vi "Get Channel.vi"(9 "name":string, 10 "Gateway IP Address (\"\": localhost)":string, 11 "Sequence Context":refnum<k7>) -> (0 "error out":errorcluster, 2 "Channel.Unit":string, 3 "Channel.Value":dbl)   [LabVIEW 2013, in "Set Channels.lvlib"]
uses:
  Set Channels.lvlib
  <vilib>/NI Veristand/Execution/Workspace/NI VeriStand - Get Single Channel Value.vi
  <vilib>/NI Veristand/Execution/Workspace/NI_VS Workspace ExecutionAPI.lvlib
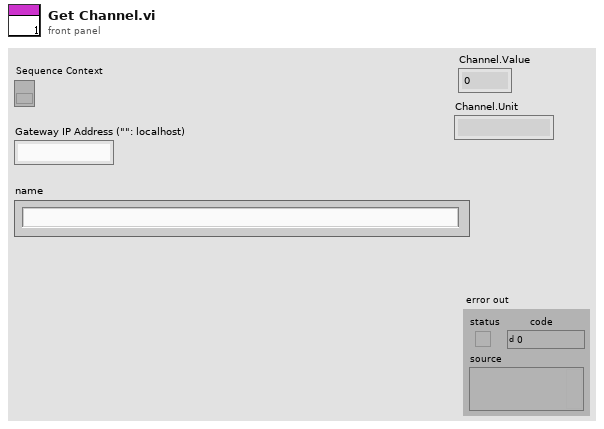
[diagram p1: front panel]
types:
  T1 = typedef "NI_VS Workspace ExecutionAPI.lvlib/WorkspaceAPI.ctl" = refnum<k24>
  T2 = typedef "NI_VS Workspace ExecutionAPI.lvlib/NodeInfo.ctl" = cluster{"Name":string, "FullPath":string, "Type":string, "IsChannel":bool, "Channel":cluster{"Unit":string, "Readable":bool, "Writable":bool, "Faultable":bool, "Scalable":bool, "RowDim":u32, "ColumnDim":u32}, "IsWaveform":bool, "Waveform":cluster{"DataType":T3}}
  T3 = typedef "NI_VS Workspace ExecutionAPI.lvlib/Waveform Data Type.ctl" = enum16{"Double", "ComplexDouble"}
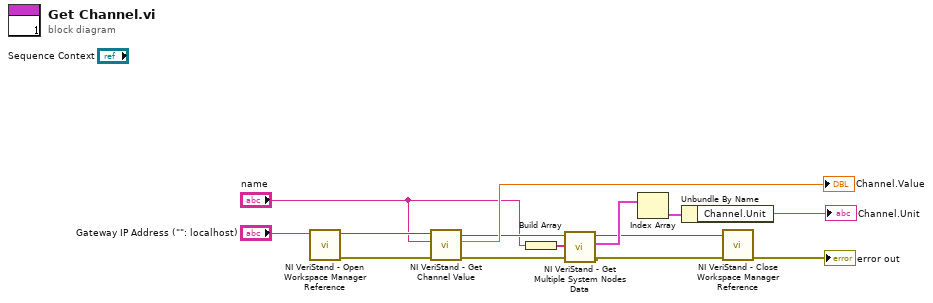
[diagram p0: block diagram]
diagram:
  n1 = call <vilib>:"NI VeriStand - Open Workspace Manager Reference.vi"("Gateway IP Address (\"\": localhost)"="Gateway IP Address (\"\": localhost)") -> ("error out"=w11:errorcluster, "WorkspaceManager"=w12:T1)  [unwired: 9 in]
  n2 = call-poly <vilib>:"NI VeriStand - Get Channel Value.vi"("error in (no error)"=w11, "Channel"="name", "WorkspaceManager in"=w12) -> ("error out"=w9:errorcluster, "Value"=→"Channel.Value":dbl, "WorkspaceManager out"=w8:T1)  [unwired: 6 in]
  n3 = Build Array("name") -> (w6:string[])
  n4 = call <vilib>:"NI VeriStand - Get Multiple System Nodes Data.vi"("error in (no error)"=w9, "Node Paths"=w6, "WorkspaceManager in"=w8) -> ("error out"=→"error out":errorcluster, "Nodes Data"=w5:T2[], "WorkspaceManager out"=w4:T1)  [unwired: 6 in]
  n5 = Index Array(array=w5) -> (element=w2:T2)  [unwired: 1 in]
  n6 = Unbundle By Name(w2) -> ("Channel.Unit"=→"Channel.Unit":string)
  n7 = call <vilib>:"NI VeriStand - Close Workspace Manager Reference.vi"("WorkspaceManager"=w4) -> ()  [unwired: 10 in, 1 out]
